vi "TTA_Set_Relay_Mode.vi"(7 "TTA COM Port":refnum<visa-resource-name>, 8 "error in":errorcluster, 11 "Mode":T1(ring)) -> (0 "error out":errorcluster)   [LabVIEW 2016]
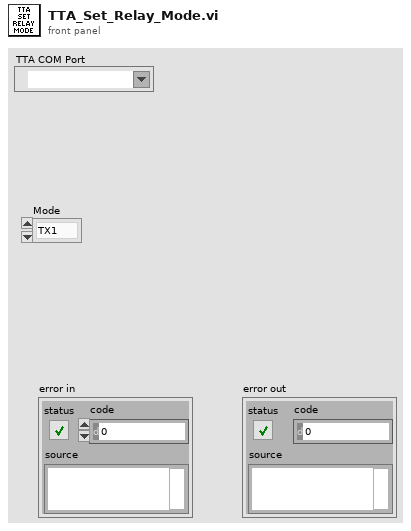
[diagram p1: front panel]
types:
  T1 = enum16{"TX1", "TX2", "TX3", "TX4", "TXx3", "TXx4", "RX1", "RX2", "RX3", "RX4", "RXx3", "RXx4", "RFCal"}
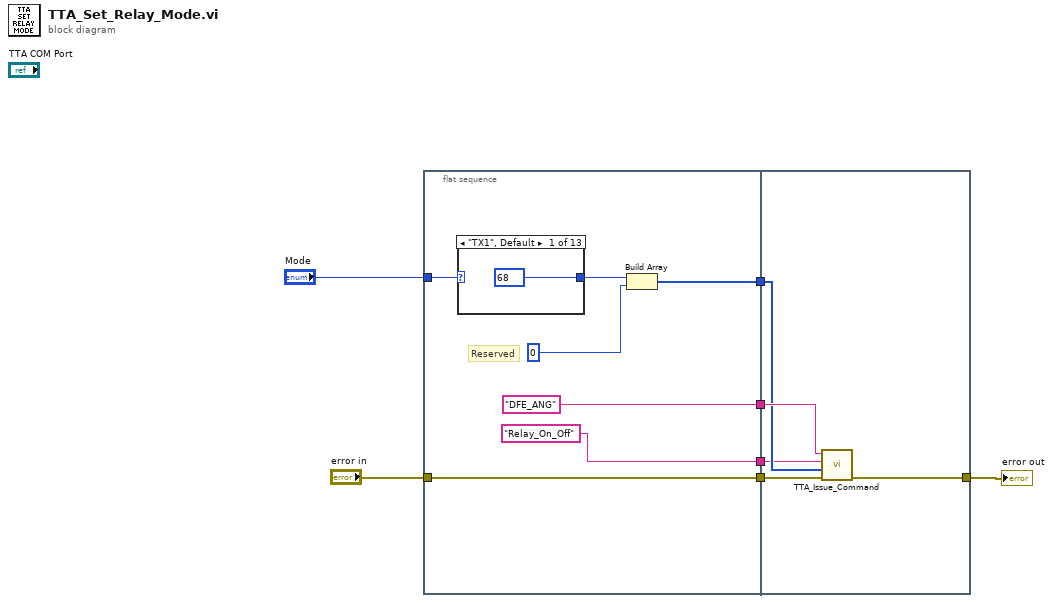
[diagram p0: block diagram]
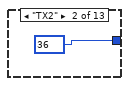
[diagram p2: hidden frame]
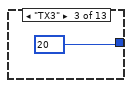
[diagram p3: hidden frame]
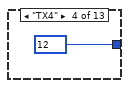
[diagram p4: hidden frame]
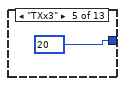
[diagram p5: hidden frame]
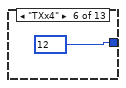
[diagram p6: hidden frame]
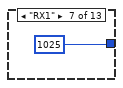
[diagram p7: hidden frame]
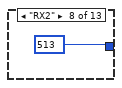
[diagram p8: hidden frame]
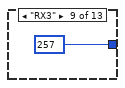
[diagram p9: hidden frame]
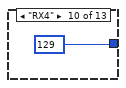
[diagram p10: hidden frame]
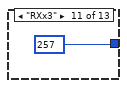
[diagram p11: hidden frame]
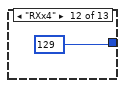
[diagram p12: hidden frame]
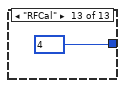
[diagram p13: hidden frame]
diagram:
  n1 = flat-sequence {
    tunnel: "Mode" -> [w14]
    tunnel: [w11] -> w6
    tunnel: [w10] -> w5
    tunnel: "error in" -> [w10]
    tunnel: ["DFE_ANG"] -> w2
    tunnel: ["Relay_On_Off"] -> w1
    tunnel: w6 -> [w29]
    tunnel: w5 -> [w32]
    tunnel: [w31] -> w4
    tunnel: w2 -> [w30]
    tunnel: w1 -> [w28]
    frame #0 {
      # "Reserved"
      n2 = case shown="\"TX1\", Default" w14 {
        tunnel: [u16 68 u16 36 u16 20 u16 12 u16 20 u16 12 u16 1025 u16 513 u16 257 u16 129 u16 257 u16 129 u16 4] -> w12
        frame "TX1", Default {
        }
        frame "TX2" {
        }
        frame "TX3" {
        }
        frame "TX4" {
        }
        frame "TXx3" {
        }
        frame "TXx4" {
        }
        frame "RX1" {
        }
        frame "RX2" {
        }
        frame "RX3" {
        }
        frame "RX4" {
        }
        frame "RXx3" {
        }
        frame "RXx4" {
        }
        frame "RFCal" {
        }
      }
      n3 = Build Array(w12, u16 0) -> (w11:u16[])
    }
    frame #1 {
      n4 = call "TTA_Issue_Command.vi"("error in"=w32, "Inputs"=w29, "SubCommand"=w28, "MainCommand"=w30) -> ("error out"=w31:errorcluster)  [unwired: 7 in]
    }
  }
  "error out" <- w4
